vi "Generate Spectra Report.vi"(11 "Measurement Information":T1={"Comments"="", "Directory Input"="", "Data file path"=path "C:/Data/EPR Data", "Scripting File"=path "C:/Data/Configuration Script.csv", "Save Data"=FALSE, "Tooth size (d11) [mm]"=0.0, "Tooth size (d12) [mm]"=0.0, "Tooth size (d21) [mm]"=0.0, "Tooth size (d22) [mm]"=0.0, "Dose of Tooth [Gy]"=0.0, "Safe Shutdown?"=FALSE, "Gases Available"=[], "Database Username"="", "Database Password"="", "Database Login URL"="", "Database Upload URL"="", "Database Success URL"="", "Database XML URL"="", "Database Resonator URL"="", "Session Number"=0, "Set #"=1, "Resonator Operator"="", "Session Type"="", "Tooth/Sample ID"="", "Volunteer ID"="", "Computer Operator"="", "Volunteer Type"="", "Site/Tooth Selection (T8,T9)"="", "Resonator"="", "Measurement Site"="", "Non-standard session?"=FALSE, "EPR DAQ Version"="", "Session Path"=path "C:/Data/EPR Data", "Chosen Applied State"="", "Chosen Initial State"="", "Time of Transition"="", "DAQ Mode"=enum."Engineering", "pO2/Scan [mmHg]"=[], "pO2/Set [mmHg]"=[], "Linewidth (HWHM)/Scan [Gauss]"=[], "Linewidth (HWHM)/Set [Gauss]"=[], "pO2 Conversion"="", "Dose Calibration Cluster"={"Dose Response"={"grand_mean"=0.0292016, "slope"=0.0188720543}, "Dose Correction"={"Sex"=1, "a0"=7.719669421, "a1"=-2.746550736, "a2"=-0.186490355, "a3"=0.041922063, "a4"=-0.849147359, "a5"=0.14330063, "a6"=0.019930219, "A_n"=40.0, "H_n"=10.12, "Dose Correction"=FALSE}, "Dose Reporting"={"Reporting is"=TRUE, "sd_threshold [AU]"=0.06, "sd_model [Gy]"=0.66, "dosimetric_threshold [Gy]"=2.0, "Add intrasession errors is"=FALSE, "Prior Radiation?"=FALSE}}, "OxyChip Slope"=0.0, "OxyChip Intercept"=0.0, "QA Mode"=enum."Select QA Mode", "QA Session?"=FALSE, "Sample Type"=enum."Empty Resonator", "Report pO2/Scan"=FALSE, "Skip End Session Save"=FALSE, "Number of sites"=enum."# Probes", "Recipient Name"="", "Sender Name"="", "Recipient Email"="", "Transition State History"=[], "pO2 Report Times"=[], "Temperature [C]"=0.0, "+Error pO2/Scan [mmHg]"=[], "-Error pO2/Scan [mmHg]"=[], "+Error pO2/Set [mmHg]"=[], "-Error pO2/Set [mmHg]"=[], "Oxy Phase Exclusion Tolerance [rad]"=0.0, "Oxy Center Exclusion Tolerance [%]"=0.0, "Oxy Exclude Unacceptable"=FALSE, "Oxy Unacceptable Estimate Flags"=[], "Save Session PPT"=FALSE, "Flagged Bad Sets"=[]} {"Oxy Center Exclusion Tolerance [%]" format="%#_9g"; "Oxy Phase Exclusion Tolerance [rad]" format="%#_9g"; "Temperature [C]" format="%#_9g"; "OxyChip Intercept" format="%#_9g"; "OxyChip Slope" format="%#_9g"; "Dose Calibration Cluster"."Dose Reporting"."dosimetric_threshold [Gy]" format="%#_9g"; "Dose Calibration Cluster"."Dose Reporting"."sd_model [Gy]" format="%#_9g"; "Dose Calibration Cluster"."Dose Reporting"."sd_threshold [AU]" format="%#_9g"; "Dose Calibration Cluster"."Dose Correction"."H_n" format="%#_9g"; "Dose Calibration Cluster"."Dose Correction"."A_n" format="%#_9g"; "Dose Calibration Cluster"."Dose Correction"."a6" format="%#.9g"; "Dose Calibration Cluster"."Dose Correction"."a5" format="%#.9g"; "Dose Calibration Cluster"."Dose Correction"."a4" format="%#.9g"; "Dose Calibration Cluster"."Dose Correction"."a3" format="%#.9g"; "Dose Calibration Cluster"."Dose Correction"."a2" format="%#.9g"; "Dose Calibration Cluster"."Dose Correction"."a1" format="%#.9g"; "Dose Calibration Cluster"."Dose Correction"."a0" format="%#.9g"; "Dose Calibration Cluster"."Dose Correction"."Sex" items=["Male"=1, "Female"=0]; "Dose Calibration Cluster"."Dose Response"."slope" format="%#_9g"; "Dose Calibration Cluster"."Dose Response"."grand_mean" format="%#_9g"}) -> (0 "error out":errorcluster)   [LabVIEW 2016]
uses:
  Types/Measurement Information.ctl
  Analysis/Dose Calculation and Reporting/Dose Calculation Control.ctl
  Types/Sample Type.ctl
panel:
  in  "PowerPoint._Application":refnum<k7>
  out "Systen\nSession\nSet":i32[](array[numeric])
  out "Spectra Graph":cluster{"B-Field":dbl[], "C-Fit":dbl[]}[](graph) caption="System: 3 || Session: 3 || Set: 3"
  # "Plotting and Saving EPR Spectra\nPlease wait..."
  # "Session Information"
  # "Oximetric Data and Information"
  # "Email"
  # "Tooth Information"
  # "Database"
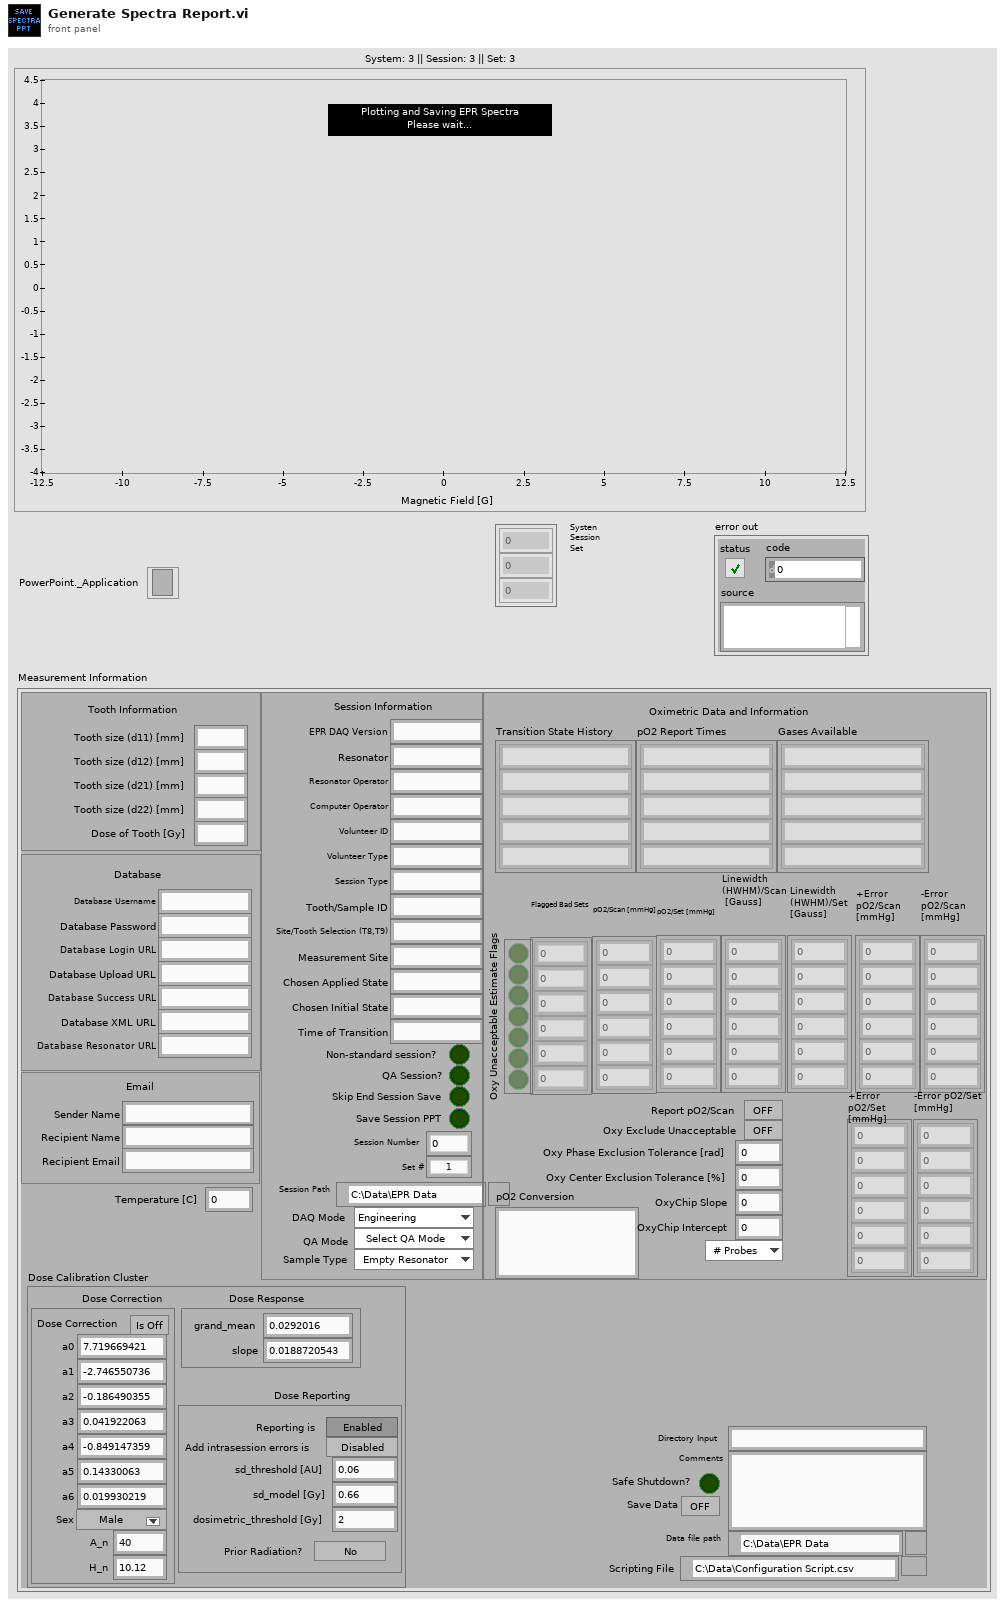
[diagram p1: front panel]
types:
  T1 = typedef "Measurement Information.ctl" = cluster{"Comments":string, "Directory Input":string, "Data file path":path, "Scripting File":path, "Save Data":bool, "Tooth size (d11) [mm]":dbl, "Tooth size (d12) [mm]":dbl, "Tooth size (d21) [mm]":dbl, "Tooth size (d22) [mm]":dbl, "Dose of Tooth [Gy]":dbl, "Safe Shutdown?":bool, "Gases Available":string[], "Database Username":string, "Database Password":string, "Database Login URL":string, "Database Upload URL":string, "Database Success URL":string, "Database XML URL":string, "Database Resonator URL":string, "Session Number":i32, "Set #":u32, "Resonator Operator":string, "Session Type":string, "Tooth/Sample ID":string, "Volunteer ID":string, "Computer Operator":string, "Volunteer Type":string, "Site/Tooth Selection (T8,T9)":string, "Resonator":string, "Measurement Site":string, "Non-standard session?":bool, "EPR DAQ Version":string, "Session Path":path, "Chosen Applied State":string, "Chosen Initial State":string, "Time of Transition":string, "DAQ Mode":enum16{"Engineering", "Dosimetry", "Oximetry"}, "pO2/Scan [mmHg]":dbl[][], "pO2/Set [mmHg]":dbl[][], "Linewidth (HWHM)/Scan [Gauss]":dbl[][], "Linewidth (HWHM)/Set [Gauss]":dbl[][], "pO2 Conversion":string, "Dose Calibration Cluster":T2, "OxyChip Slope":dbl, "OxyChip Intercept":dbl, "QA Mode":enum16{"Select QA Mode", "QA-Start/End", "QA-Mid", "QA-Weekly", "QA-Eng", "Check Calibration"}, "QA Session?":bool, "Sample Type":T3, "Report pO2/Scan":bool, "Skip End Session Save":bool, "Number of sites":enum16{"# Probes", "1", "2", "3", "4"}, "Recipient Name":string, "Sender Name":string, "Recipient Email":string, "Transition State History":string[], "pO2 Report Times":string[], "Temperature [C]":dbl, "+Error pO2/Scan [mmHg]":dbl[][], "-Error pO2/Scan [mmHg]":dbl[][], "+Error pO2/Set [mmHg]":dbl[][], "-Error pO2/Set [mmHg]":dbl[][], "Oxy Phase Exclusion Tolerance [rad]":dbl, "Oxy Center Exclusion Tolerance [%]":dbl, "Oxy Exclude Unacceptable":bool, "Oxy Unacceptable Estimate Flags":bool[], "Save Session PPT":bool, "Flagged Bad Sets":u32[]}
  T2 = typedef "Dose Calculation Control.ctl" = cluster{"Dose Response":cluster{"grand_mean":dbl, "slope":dbl}, "Dose Correction":cluster{"Sex":u16, "a0":dbl, "a1":dbl, "a2":dbl, "a3":dbl, "a4":dbl, "a5":dbl, "a6":dbl, "A_n":dbl, "H_n":dbl, "Dose Correction":bool}, "Dose Reporting":cluster{"Reporting is":bool, "sd_threshold [AU]":dbl, "sd_model [Gy]":dbl, "dosimetric_threshold [Gy]":dbl, "Add intrasession errors is":bool, "Prior Radiation?":bool}}
  T3 = typedef "Sample Type.ctl" = enum16{"Empty Resonator", "IRS", "BallZero", "Irradiated Tooth", "Non-irradiated Tooth", "OxyChip", "LiPc", "PDT", "India Ink"}
  T4 = cluster{"B-Field":dbl[], "In-Phase EPR Scan":dbl[]}
  T5 = cluster{"Header":string, "B-Field":dbl[], "In-Phase EPR Scan":dbl[], "Out-Phase EPR Scan":dbl[], "Balance":dbl[], "Phase Error":dbl[], "AFC Error":dbl[], "Out-Phase EPR Median":dbl[], "In-Phase EPR Median":dbl[], "C-Fit":dbl[], "C-Fit NoBaseline":dbl[], "Modulation Amplitude [G]":dbl, "Modulation Frequency [Hz]":dbl, "Model":string}
  T6 = cluster{"B-Field":dbl[], "In-Phase EPR Median":dbl[]}
  T7 = cluster{"B-Field":dbl[], "In-Phase EPR Scan":dbl[]}[]
  T8 = cluster{"B-Field":dbl[], "In-Phase EPR Median":dbl[]}[]
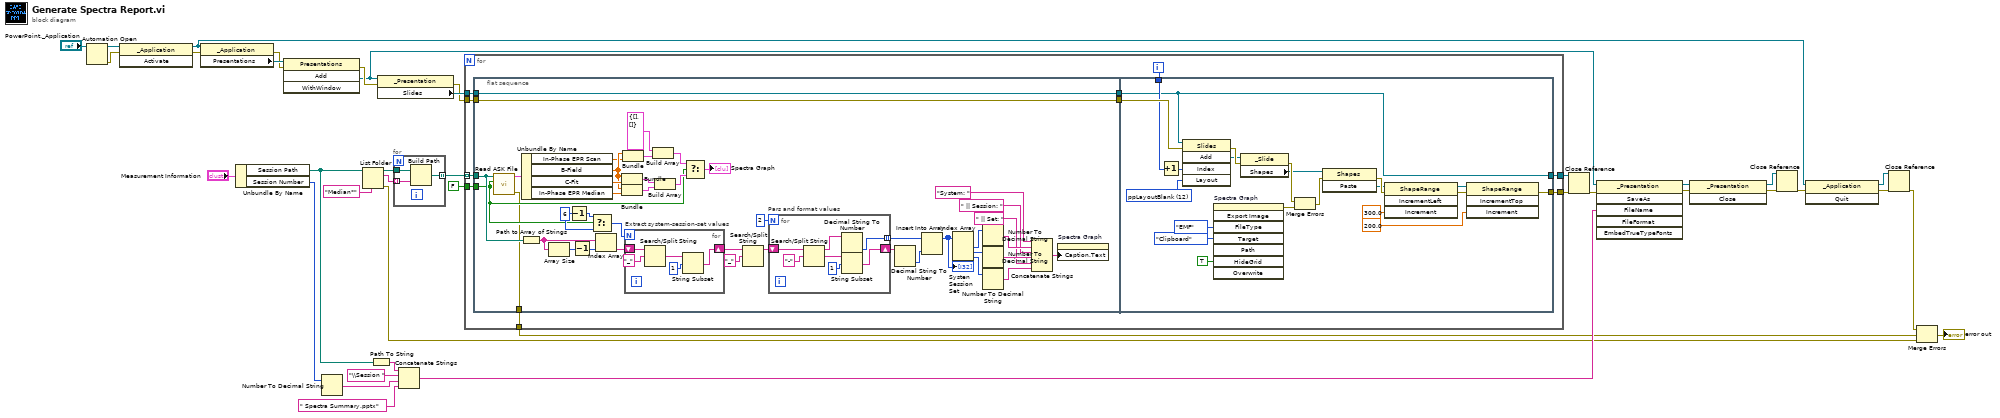
[diagram p0: block diagram]
diagram:
  n1 = Automation Open(Automation Refnum="PowerPoint._Application") -> (Automation Refnum=w37:refnum<k7>, error out=w36:errorcluster)  [unwired: 3 in]
  n2 = invoke class="_Application" method="Activate"(reference=w37, error in=w36) -> (reference out=w20:refnum<k7>, error out=w35:errorcluster)  [unwired: 1 in, 1 out]
  n3 = property class="_Application"(reference=w20, error in=w35) -> (error out=w33:errorcluster, "Presentations"=w34:refnum<k7>)  [unwired: 1 out]
  n4 = Unbundle By Name("Measurement Information") -> ("Session Path"=w10:path, "Session Number"=w9:i32)
  n5 = invoke class="Presentations" method="Add"(reference=w34, error in=w33) -> (error out=w32:errorcluster, "Add"=w25:refnum<k7>)  [unwired: 2 in, 2 out]
  n6 = Number To Decimal String(number=w9) -> (decimal integer string=w13:string)  [unwired: 1 in]
  n7 = List Folder(path=w10, pattern="Median*") -> (path out=w28:path, filenames=w29:string[], error out=w4:errorcluster)  [unwired: 2 in, 1 out]
  n8 = Path To String(path=w10) -> (string=w15:string)
  n9 = property class="_Presentation"(reference=w25, error in=w32) -> (error out=w30:errorcluster, "Slides"=w31:refnum<k7>)  [unwired: 1 out]
  n10 = for {
    tunnel: w28 -> [w41]
    tunnel: w29 -> [w40] mode=indexing
    tunnel: [w39] -> w26 mode=indexing
    n11 = Build Path(base path=w41, name or relative path=w40) -> (appended path=w39:path)
  }
  n12 = Concatenate Strings(w15, "\\Session " ("string"), w13, " Spectra Summary.pptx" ("FileName")) -> (w16:string)
  n13 = for {
    tunnel: w26 -> [w49] mode=indexing
    tunnel: FALSE ("Scan (T) / Median (F)") -> [w48]
    tunnel: w31 -> [w47]
    tunnel: w30 -> [w46]
    tunnel: [w44] -> w24
    tunnel: [w43] -> w22
    tunnel: [w42] -> w1
    i -> [w45]
    n14 = flat-sequence {
      tunnel: [w54] -> w51
      tunnel: [w53] -> w50
      tunnel: w49 -> [w56]
      tunnel: w48 -> [w55]
      tunnel: w47 -> [w54]
      tunnel: w46 -> [w53]
      tunnel: [w52] -> w42
      tunnel: w51 -> [w108]
      tunnel: w50 -> [w110]
      tunnel: w45 -> [w109]
      tunnel: [w108] -> w44
      tunnel: [w107] -> w43
      frame #0 {
        w81 = 6
        n15 = call "Read ASK File.vi"("Scan (T) / Median (F)"=w55, "File Path"=w56) -> ("error out"=w52:errorcluster, "Data Cluster Out"=w93:T5)  [unwired: 8 in]
        n16 = Path to Array of Strings(0:w56) -> (2:w87:string[])  [unwired: 1 out]
        n17 = Unbundle By Name(w93) -> ("In-Phase EPR Scan"=w62:dbl[], "B-Field"=w63:dbl[], "C-Fit"=w92:dbl[], "In-Phase EPR Median"=w91:dbl[])
        n18 = Array Size(array=w87) -> (size(s)=w88:i32)
        n19 = Decrement(x=w81) -> (x-1=w82:i32)
        n20 = Decrement(x=w88) -> (x-1=w86:i32)
        n21 = Select(t=w82, s=w55, f=w81) -> (s? t:f=w80:i32)
        n22 = Index Array(array=w87, index=w86) -> (element=w85:string)
        n23 = Bundle("B-Field"=w63, "C-Fit"=w92) -> (w90:cluster{"B-Field":dbl[], "C-Fit":dbl[]})  [unwired: 1 in]
        n24 = Bundle("B-Field"=w63, "In-Phase EPR Median"=w91) -> (w89:T6)  [unwired: 1 in]
        n25 = Bundle("B-Field"=w63, "In-Phase EPR Scan"=w62) -> (w58:T4)  [unwired: 1 in]
        n26 = for "Extract system-session-set values" {
          N: w80 -> [_]
          shift-right: [w101] -> w83
          shift-left: w85 -> [w104]
          n27 = Search/Split String(string=w104, search string/char (-)="_") -> (match + rest of string=w103:string)  [unwired: 1 in, 2 out]
          n28 = String Subset(string=w103, offset (0)=1) -> (substring=w101:string)  [unwired: 1 in]
        }
        n29 = Build Array(T4 {"B-Field"=[], "In-Phase EPR Scan"=[]} ("element"), w58) -> (w60:T7)
        n30 = Build Array(w90, w89) -> (w61:T8)
        n31 = Select(t=w60, s=w55, f=w61) -> (s? t:f=→"Spectra Graph":T8)
        n32 = Search/Split String(string=w83, search string/char (-)="_") -> (substring before match=w78:string)  [unwired: 1 in, 2 out]
        n33 = for "Pars and format values" {
          N: 2 -> [_]
          shift-right: [w96] -> w77
          shift-left: w78 -> [w99]
          tunnel: [w94] -> w76 mode=indexing
          n34 = Search/Split String(string=w99, search string/char (-)="-") -> (substring before match=w95:string, match + rest of string=w98:string)  [unwired: 1 in, 1 out]
          n35 = Decimal String To Number(string=w95) -> (number=w94:i32)  [unwired: 2 in, 1 out]
          n36 = String Subset(string=w98, offset (0)=1) -> (substring=w96:string)  [unwired: 1 in]
        }
        n37 = Decimal String To Number(string=w77) -> (number=w75:i32)  [unwired: 2 in, 1 out]
        n38 = Insert Into Array(array=w76, new element=w75) -> (w73:i32[])  [unwired: 1 in]
        "Systen\nSession\nSet" <- w73
        n39 = Index Array(array=w73) -> (element #1=w72:i32, element #2=w71:i32, element #3=w70:i32)  [unwired: 3 in]
        n40 = Number To Decimal String(number=w72) -> (decimal integer string=w69:string)  [unwired: 1 in]
        n41 = Number To Decimal String(number=w71) -> (decimal integer string=w67:string)  [unwired: 1 in]
        n42 = Number To Decimal String(number=w70) -> (decimal integer string=w65:string)  [unwired: 1 in]
        n43 = Concatenate Strings("System: " ("string"), w69, " || Session: " ("string"), w67, " || Set: " ("string"), w65) -> (w64:string)
        n44 = property on="Spectra Graph" class="XYGraph (strict)"("Caption.Text"=w64) -> ()  [unwired: 2 in, 2 out]
      }
      frame #1 {
        w111 = 12 items=["ppLayoutMixed"=-2, "ppLayoutTitle"=1, "ppLayoutText"=2, "ppLayoutTwoColumnText"=3, "ppLayoutTable"=4, "ppLayoutTextAndChart"=5, "ppLayoutChartAndText"=6, "ppLayoutOrgchart"=7, "ppLayoutChart"=8, "ppLayoutTextAndClipart"=9, "ppLayoutClipartAndText"=10, "ppLayoutTitleOnly"=11, "ppLayoutBlank"=12, "ppLayoutTextAndObject"=13, "ppLayoutObjectAndText"=14, "ppLayoutLargeObject"=15, "ppLayoutObject"=16, "ppLayoutTextAndMediaClip"=17, "ppLayoutMediaClipAndText"=18, "ppLayoutObjectOverText"=19, "ppLayoutTextOverObject"=20, "ppLayoutTextAndTwoObjects"=21, "ppLayoutTwoObjectsAndText"=22, "ppLayoutTwoObjectsOverText"=23, "ppLayoutFourObjects"=24, "ppLayoutVerticalText"=25, "ppLayoutClipArtAndVerticalText"=26, "ppLayoutVerticalTitleAndText"=27, "ppLayoutVerticalTitleAndTextOverChart"=28, "ppLayoutTwoObjects"=29, "ppLayoutObjectAndTwoObjects"=30, "ppLayoutTwoObjectsAndObject"=31, "ppLayoutCustom"=32, "ppLayoutSectionHeader"=33, "ppLayoutComparison"=34, "ppLayoutContentWithCaption"=35, "ppLayoutPictureWithCaption"=36] ("Layout")
        n45 = Increment(x=w109) -> (x+1=w123:i32)
        n46 = invoke class="Slides" method="Add"(reference=w108, error in=w110, "Index"=w123, "Layout"=w111) -> (error out=w117:errorcluster, "Add"=w115:refnum<k7>)  [unwired: 1 in, 3 out]
        n47 = invoke on="Spectra Graph" class="XYGraph (strict)" method="Export Image"("FileType"=enum32{"BMP", "EPS", "EMF", "PICT"}."EMF" ("File Type"), "Target"=enum32{"File", "Clipboard"}."Clipboard", "HideGrid"=TRUE ("Hide Grid")) -> (error out=w126:errorcluster)  [unwired: 5 in, 7 out]
        n48 = property class="_Slide"(reference=w115, error in=w117) -> (error out=w124:errorcluster, "Shapes"=w116:refnum<k7>)  [unwired: 1 out]
        n49 = Merge Errors(w124, w126) -> (w125:errorcluster)
        n50 = invoke class="Shapes" method="Paste"(reference=w116, error in=w125) -> (error out=w122:errorcluster, "Paste"=w118:refnum<k7>)  [unwired: 1 in, 1 out]
        n51 = invoke class="ShapeRange" method="IncrementLeft"(reference=w118, error in=w122, "Increment"=sgl 300.0 ("Left")) -> (reference out=w119:refnum<k7>, error out=w120:errorcluster)  [unwired: 1 in, 2 out]
        n52 = invoke class="ShapeRange" method="IncrementTop"(reference=w119, error in=w120, "Increment"=sgl 200.0) -> (error out=w107:errorcluster)  [unwired: 1 in, 3 out]
      }
    }
  }
  n53 = Close Reference(reference=w24, error in (no error)=w22) -> (error out=w23:errorcluster)
  n54 = invoke class="_Presentation" method="SaveAs"(reference=w25, error in=w23, "FileName"=w16) -> (reference out=w8:refnum<k7>, error out=w7:errorcluster)  [unwired: 3 in, 4 out]
  n55 = invoke class="_Presentation" method="Close"(reference=w8, error in=w7) -> (reference out=w6:refnum<k7>, error out=w5:errorcluster)  [unwired: 1 in, 1 out]
  n56 = Close Reference(reference=w6, error in (no error)=w5) -> (error out=w18:errorcluster)
  n57 = invoke class="_Application" method="Quit"(reference=w20, error in=w18) -> (reference out=w19:refnum<k7>, error out=w21:errorcluster)  [unwired: 1 in, 1 out]
  n58 = Close Reference(reference=w19, error in (no error)=w21) -> (error out=w3:errorcluster)
  n59 = Merge Errors(w3, w1, w4) -> (→"error out":errorcluster)
